vi "test_get_ROI_boundary.vi"() -> ()   [LabVIEW 2010]
uses:
  point_cluster.ctl
  <vilib>/vision/Image Controls.llb/IMAQ Image.ctl
  <vilib>/vision/NI_Vision_Development_Module.lvlib
panel:
  out "XY Graph":cluster{"x":i32, "y":i32}[](graph)
  out "Labelled":T1(plugin-control)
  in  "Threshold Values":T2(slide)={"Minimum Value"=0.0, "Maximum Value"=155.0} scale=0.0..255.0
  in  "stop":bool
  in  "load button":bool
  out "Image":T1(plugin-control)
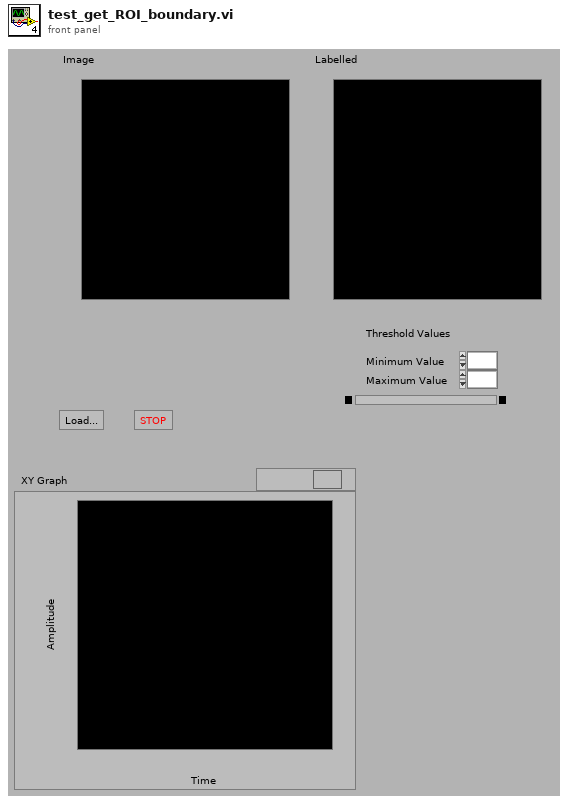
[diagram p1: front panel]
types:
  T1 = typedef "IMAQ Image.ctl" = refnum<image>
  T2 = cluster{"Minimum Value":sgl, "Maximum Value":sgl}
  T3 = typedef "point_cluster.ctl" = cluster{"x":i32, "y":i32}
  T4 = enum32{"AutoM", "Close", "Dilate", "Erode", "Gradient", "Gradient out", "Gradient in", "Hit miss", "Open", "PClose", "POpen", "Thick", "Thin"}
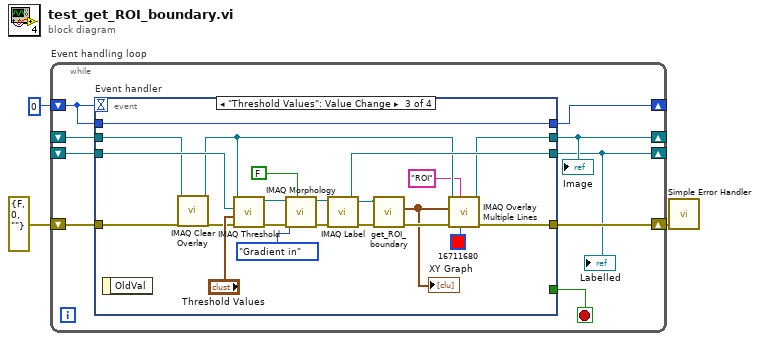
[diagram p0: block diagram]
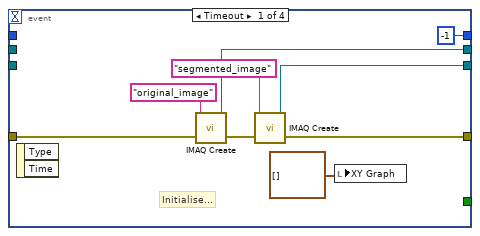
[diagram p2: hidden frame]
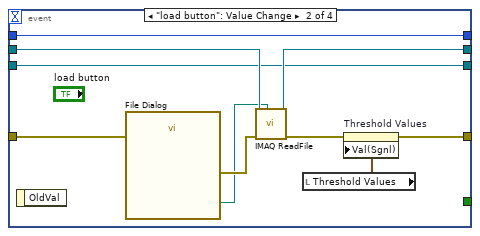
[diagram p3: hidden frame]
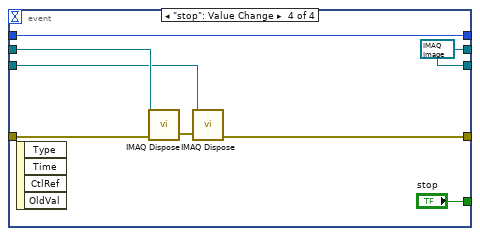
[diagram p4: hidden frame]
diagram:
  n1 = while "Event handling loop" {
    shift-right: [w9] -> w1
    shift-left: errorcluster {"status"=FALSE, "code"=0, "source"=""} ("error in (no error)") -> [w12]
    shift-right: [w10] -> _
    shift-left: 0 -> [w11]
    shift-right: [w7] -> _
    shift-left: _ -> [w8]
    shift-right: [w4] -> _
    shift-left: _ -> [w5]
    stop <- w6 stop-if-true
    n2 = event "Event handler" shown="[2] \"Threshold Values\": Value Change" {
      selector: _ -> [_ _ _ _]
      dyn-events: _ -> [_ _ _ _]
      timeout: w11 -> [_ _ _ _]
      tunnel: w12 -> [w20 w31 w38 w57]
      tunnel: w11 -> [_ w30 w52 w60]
      tunnel: [-1 w30 w52 w60] -> w10
      tunnel: [w16 w23 w41 w56] -> w9
      tunnel: [w18 w27 w40 w53] -> w7
      tunnel: w8 -> [_ w28 w36 w55]
      tunnel: [_ _ _ "stop"] -> w6
      tunnel: w5 -> [_ w25 w47 w54]
      tunnel: [w15 w25 w43 w53] -> w4
      event Timeout {
        # "Initialise..."
        n3 = event-data() -> ()  [unwired: 1 in, 2 out]
        n4 = call "IMAQ Create"("Image Name"="original_image", "error in (no error)"=w20) -> ("New Image"=w18:T1, "error out"=w17:errorcluster)  [unwired: 3 in]
        n5 = call "IMAQ Create"("Image Name"="segmented_image", "error in (no error)"=w17) -> ("New Image"=w15:T1, "error out"=w16:errorcluster)  [unwired: 3 in]
        n6 = local write "XY Graph"(T3[] []) -> ()
      }
      event "load button": Value Change {
        n7 = event-data() -> ()  [unwired: 1 in, 1 out]
        n8 = call "File Dialog"("error in"=w31) -> ("selected path"=w26:path, "error out"=w29:errorcluster)  [unwired: 11 in, 2 out]
        n9 = call "IMAQ ReadFile"("File Path"=w26, "error in (no error)"=w29, "Image"=w28) -> ("error out"=w24:errorcluster, "Image Out"=w27:T1)  [unwired: 4 in, 3 out]
        n10 = local read "Threshold Values"() -> (w22:T2)
        n11 = property on="Threshold Values" class="Slide (strict)"(error in=w24, "Val(Sgnl)"=w22) -> (error out=w23:errorcluster)  [unwired: 1 in, 1 out]
      }
      event "Threshold Values": Value Change {
        n12 = event-data() -> ()  [unwired: 1 in, 1 out]
        n13 = call "IMAQ Clear Overlay"("error in (no error)"=w38, "Image"=w36) -> ("error out"=w37:errorcluster, "Image Out"=w35:T1)  [unwired: 8 in]
        n14 = call "IMAQ Threshold"("error in (no error)"=w37, "Range"="Threshold Values", "Image Dst"=w47, "Image Src"=w35) -> ("error out"=w51:errorcluster, "Image Dst Out"=w50:T1)  [unwired: 6 in]
        n15 = call "IMAQ Morphology"("Square/Hexa (Square)"=FALSE, "error in (no error)"=w51, "Operation"=T4."Gradient in", "Image Src"=w50) -> ("error out"=w46:errorcluster, "Image Dst Out"=w45:T1)  [unwired: 3 in, 3 out]
        n16 = call "IMAQ Label"("error in (no error)"=w46, "Image Src"=w45) -> ("error out"=w44:errorcluster, "Image Dst Out"=w43:T1)  [unwired: 2 in, 1 out]
        n17 = call "get_ROI_boundary.vi"("error in (no error)"=w44, "image in"=w43) -> ("error out"=w42:errorcluster, "points"=w33:T3[])  [unwired: 8 in]
        "XY Graph" <- w33
        n18 = call "IMAQ Overlay Multiple Lines"("Color"=u32 16711680, "Group"="ROI", "error in (no error)"=w42, "Line End Points"=w33, "Image"=w35) -> ("error out"=w41:errorcluster, "Image Out"=w40:T1)  [unwired: 5 in]
      }
      event "stop": Value Change {
        w53 = T1 refnum ("Image Out")
        n19 = event-data() -> ()  [unwired: 1 in, 4 out]
        n20 = call "IMAQ Dispose"("Image"=w55, "error in (no error)"=w57) -> ("error out"=w58:errorcluster)  [unwired: 1 in, 3 out]
        n21 = call "IMAQ Dispose"("Image"=w54, "error in (no error)"=w58) -> ("error out"=w56:errorcluster)  [unwired: 1 in, 3 out]
      }
    }
    "Image" <- w7
    "Labelled" <- w4
  }
  n22 = call <vilib>:"Simple Error Handler.vi"("error in (no error)"=w1) -> ()  [unwired: 4 in, 5 out]
